vi "upload.part_core.vi"(8 "error in":errorcluster, 9 "Body":string, 10 "Full Path":string, 11 "REST Client":refnum<class "REST Client.lvclass">) -> (0 "error out":errorcluster, 2 "Response":string)   [LabVIEW 2020, in "Multipart Upload.lvclass"]
uses:
  Nominal Client MultiPart Upload/Multipart Upload.lvclass
  <vilib>/addons/_JKI.lib/REST Client/classes/REST Client/REST Client.lvclass
  error.vi
  trace.payload_sent.vi
  trace.payload_received.vi
  error.vi/859f8e04-e495-489b-b5b4-7ac163f56130.vi
  trace.generate.vi
  <vilib>/AdvancedString/1D String Array to Delimited String.vi
  <vilib>/JDP Science/JDP Science Common Utilities/Trim Whitespace__JDP.vi
  trace.calling_method.vi
  <vilib>/Utility/libraryn.llb/Get File Extension.vi
  log_file.write.vi
  <vilib>/JDP Science/JSONtext/Get all Object Items.vi
  <vilib>/Utility/error.llb/Error Cluster From Error Code.vi
  <vilib>/JDP Science/JSONtext/JSON text to Variant.vi
  <vilib>/JDP Science/JSONtext/LVClass Serializer/JSONtext LVClass Serializer.lvclass
  <vilib>/addons/_JKI.lib/REST Client/classes/Response Headers/Response Headers.lvclass
  Nominal Client.lvclass
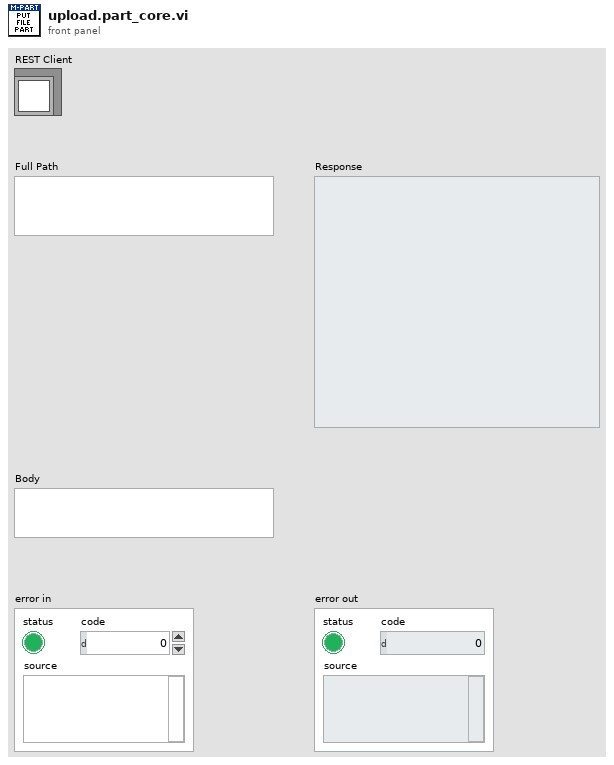
[diagram p1: front panel]
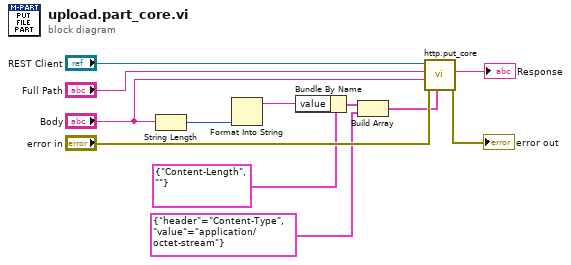
[diagram p0: block diagram]
diagram:
  n1 = String Length(string="Body") -> (length=w4:i32)
  n2 = Format Into String(w4) -> (resulting string=w3:string)  [unwired: 3 in, 1 out]
  n3 = Bundle By Name(cluster=cluster{"header":string, "value":string} {"header"="Content-Length", "value"=""} ("Header"), "value"=w3) -> (w6:cluster{"header":string, "value":string})
  n4 = Build Array(w6, cluster{"header":string, "value":string} {"header"="Content-Type", "value"="application/octet-stream"} ("Header")) -> (w5:cluster{"header":string, "value":string}[])
  n5 = call "http.put_core.vi"("specific headers in"=w5, "error in"="error in", "Body"="Body", "Path"="Full Path", "REST Client"="REST Client") -> ("error out"=→"error out":errorcluster, "Response"=→"Response":string)  [unwired: 4 in, 1 out]
